vi "Copy To Memory-User.vi"(6 "Select User Trace (1: 1)":u16(ring)=1 items=["1"=1, "2"=2, "3"=3, "4"=4, "5"=5, "6"=6, "7"=7, "8"=8], 7 "Select Current Trace (1: 1)":u16(ring)=1 items=["1"=1, "2"=2, "3"=3, "4"=4, "5"=5, "6"=6, "7"=7, "8"=8], 8 "error in (no error)":errorcluster, 9 "Operation (0: Copy To Memory)":enum16{"Copy To Memory", "Copy To User"}(ring), 10 "Measurement Type (6: Phase Noise)":u16(ring)=6 items=["AM Noise"=1, "Baseband Noise"=2, "Freq/Power"=3, "Spectrum"=4, "Transient"=5, "Phase Noise"=6, "User"=7], 11 "VISA resource name":refnum<visa-resource-name>) -> (0 "error out":errorcluster, 3 "VISA resource name out":refnum<visa-resource-name>)   [LabVIEW 2011, in "Agilent E5052X.lvlib"]
doc: "Copies the selected trace to memory or to the selected user trace."
uses:
  Agilent E5052X.lvlib
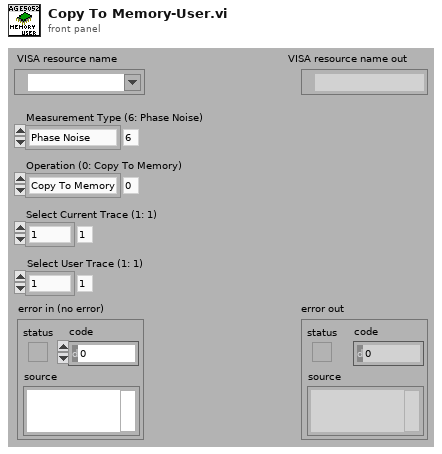
[diagram p1: front panel]
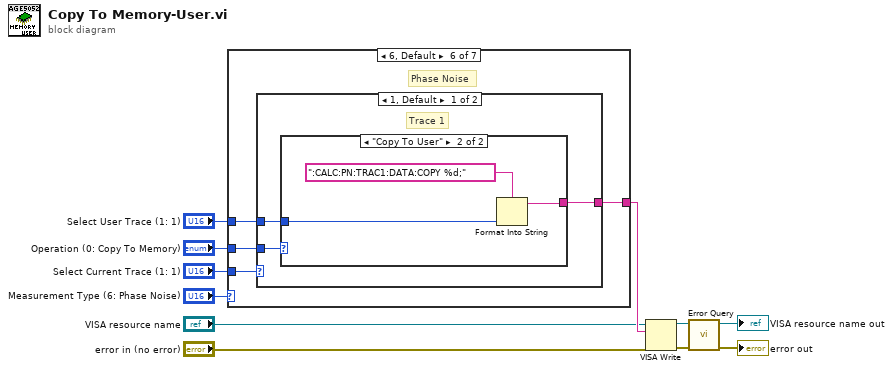
[diagram p0: block diagram]
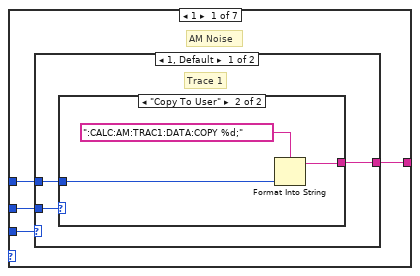
[diagram p2: hidden frame]
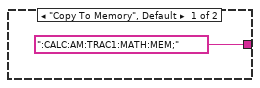
[diagram p3: hidden frame]
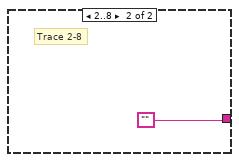
[diagram p4: hidden frame]
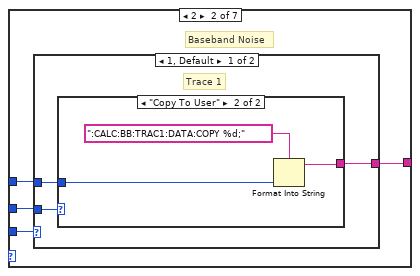
[diagram p5: hidden frame]
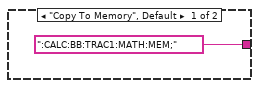
[diagram p6: hidden frame]
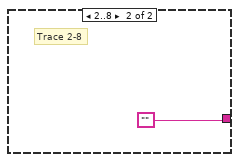
[diagram p7: hidden frame]
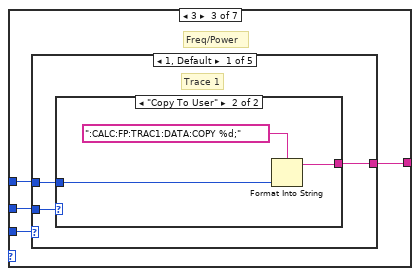
[diagram p8: hidden frame]
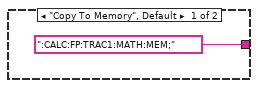
[diagram p9: hidden frame]
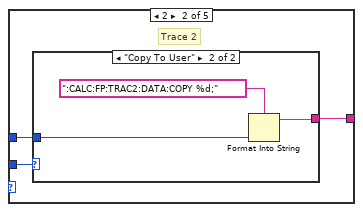
[diagram p10: hidden frame]
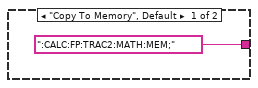
[diagram p11: hidden frame]
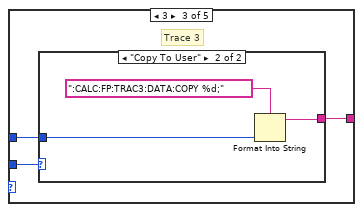
[diagram p12: hidden frame]
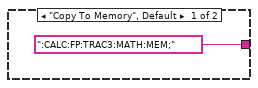
[diagram p13: hidden frame]
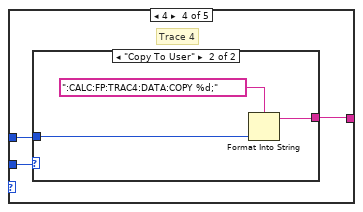
[diagram p14: hidden frame]
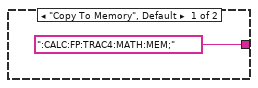
[diagram p15: hidden frame]
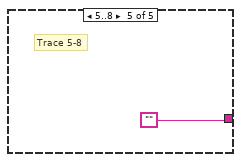
[diagram p16: hidden frame]
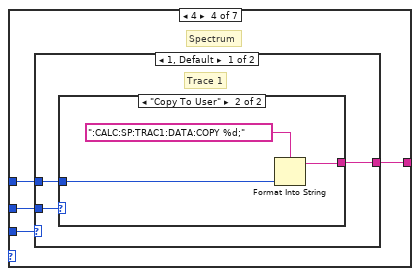
[diagram p17: hidden frame]
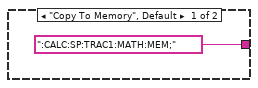
[diagram p18: hidden frame]
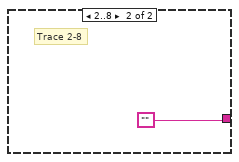
[diagram p19: hidden frame]
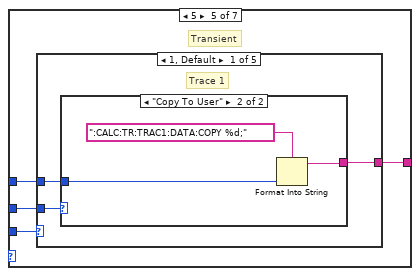
[diagram p20: hidden frame]
diagram:
  n1 = case shown="6, Default" "Measurement Type (6: Phase Noise)" {
    tunnel: "Select Current Trace (1: 1)" -> [w15 w25 w37 w70 w82 w115 w127]
    tunnel: "Operation (0: Copy To Memory)" -> [w14 w26 w38 w71 w83 w116 w128]
    tunnel: "Select User Trace (1: 1)" -> [w13 w27 w39 w72 w84 w117 w129]
    tunnel: [w12 w24 w36 w69 w81 w114 w126] -> w8
    frame 1 {
      # "AM Noise"
      n2 = case shown="1, Default" w15 {
        tunnel: w14 -> [w18 _]
        tunnel: w13 -> [w17 _]
        tunnel: [w16 ""] -> w12
        frame 1, Default {
          # "Trace 1"
          n3 = case shown="\"Copy To User\"" w18 {
            tunnel: [":CALC:AM:TRAC1:MATH:MEM;" w20] -> w16
            tunnel: w17 -> [_ w22]
            frame "Copy To Memory", Default {
            }
            frame "Copy To User" {
              n4 = Format Into String(format string=":CALC:AM:TRAC1:DATA:COPY %d;", w22) -> (resulting string=w20:string)  [unwired: 2 in, 1 out]
            }
          }
        }
        frame 2..8 {
          # "Trace 2-8"
        }
      }
    }
    frame 2 {
      # "Baseband Noise"
      n5 = case shown="1, Default" w25 {
        tunnel: w26 -> [w30 _]
        tunnel: w27 -> [w29 _]
        tunnel: [w28 ""] -> w24
        frame 1, Default {
          # "Trace 1"
          n6 = case shown="\"Copy To User\"" w30 {
            tunnel: [":CALC:BB:TRAC1:MATH:MEM;" w32] -> w28
            tunnel: w29 -> [_ w34]
            frame "Copy To Memory", Default {
            }
            frame "Copy To User" {
              n7 = Format Into String(format string=":CALC:BB:TRAC1:DATA:COPY %d;", w34) -> (resulting string=w32:string)  [unwired: 2 in, 1 out]
            }
          }
        }
        frame 2..8 {
          # "Trace 2-8"
        }
      }
    }
    frame 3 {
      # "Freq/Power"
      n8 = case shown="1, Default" w37 {
        tunnel: w38 -> [w42 w48 w55 w62 _]
        tunnel: w39 -> [w41 w49 w56 w63 _]
        tunnel: [w40 w47 w54 w61 ""] -> w36
        frame 1, Default {
          # "Trace 1"
          n9 = case shown="\"Copy To User\"" w42 {
            tunnel: [":CALC:FP:TRAC1:MATH:MEM;" w44] -> w40
            tunnel: w41 -> [_ w46]
            frame "Copy To Memory", Default {
            }
            frame "Copy To User" {
              n10 = Format Into String(format string=":CALC:FP:TRAC1:DATA:COPY %d;", w46) -> (resulting string=w44:string)  [unwired: 2 in, 1 out]
            }
          }
        }
        frame 2 {
          # "Trace 2"
          n11 = case shown="\"Copy To User\"" w48 {
            tunnel: [":CALC:FP:TRAC2:MATH:MEM;" w51] -> w47
            tunnel: w49 -> [_ w53]
            frame "Copy To Memory", Default {
            }
            frame "Copy To User" {
              n12 = Format Into String(format string=":CALC:FP:TRAC2:DATA:COPY %d;", w53) -> (resulting string=w51:string)  [unwired: 2 in, 1 out]
            }
          }
        }
        frame 3 {
          # "Trace 3"
          n13 = case shown="\"Copy To User\"" w55 {
            tunnel: [":CALC:FP:TRAC3:MATH:MEM;" w58] -> w54
            tunnel: w56 -> [_ w60]
            frame "Copy To Memory", Default {
            }
            frame "Copy To User" {
              n14 = Format Into String(format string=":CALC:FP:TRAC3:DATA:COPY %d;", w60) -> (resulting string=w58:string)  [unwired: 2 in, 1 out]
            }
          }
        }
        frame 4 {
          # "Trace 4"
          n15 = case shown="\"Copy To User\"" w62 {
            tunnel: [":CALC:FP:TRAC4:MATH:MEM;" w65] -> w61
            tunnel: w63 -> [_ w67]
            frame "Copy To Memory", Default {
            }
            frame "Copy To User" {
              n16 = Format Into String(format string=":CALC:FP:TRAC4:DATA:COPY %d;", w67) -> (resulting string=w65:string)  [unwired: 2 in, 1 out]
            }
          }
        }
        frame 5..8 {
          # "Trace 5-8"
        }
      }
    }
    frame 4 {
      # "Spectrum"
      n17 = case shown="1, Default" w70 {
        tunnel: w71 -> [w75 _]
        tunnel: w72 -> [w74 _]
        tunnel: [w73 ""] -> w69
        frame 1, Default {
          # "Trace 1"
          n18 = case shown="\"Copy To User\"" w75 {
            tunnel: [":CALC:SP:TRAC1:MATH:MEM;" w77] -> w73
            tunnel: w74 -> [_ w79]
            frame "Copy To Memory", Default {
            }
            frame "Copy To User" {
              n19 = Format Into String(format string=":CALC:SP:TRAC1:DATA:COPY %d;", w79) -> (resulting string=w77:string)  [unwired: 2 in, 1 out]
            }
          }
        }
        frame 2..8 {
          # "Trace 2-8"
        }
      }
    }
    frame 5 {
      # "Transient"
      n20 = case shown="1, Default" w82 {
        tunnel: w83 -> [w87 w93 w100 w107 _]
        tunnel: w84 -> [w86 w94 w101 w108 _]
        tunnel: [w85 w92 w99 w106 ""] -> w81
        frame 1, Default {
          # "Trace 1"
          n21 = case shown="\"Copy To User\"" w87 {
            tunnel: [":CALC:TR:TRAC1:MATH:MEM;" w89] -> w85
            tunnel: w86 -> [_ w91]
            frame "Copy To Memory", Default {
            }
            frame "Copy To User" {
              n22 = Format Into String(format string=":CALC:TR:TRAC1:DATA:COPY %d;", w91) -> (resulting string=w89:string)  [unwired: 2 in, 1 out]
            }
          }
        }
        frame 2 {
          # "Trace 2"
          n23 = case shown="\"Copy To User\"" w93 {
            tunnel: [":CALC:TR:TRAC2:MATH:MEM;" w96] -> w92
            tunnel: w94 -> [_ w98]
            frame "Copy To Memory", Default {
            }
            frame "Copy To User" {
              n24 = Format Into String(format string=":CALC:TR:TRAC2:DATA:COPY %d;", w98) -> (resulting string=w96:string)  [unwired: 2 in, 1 out]
            }
          }
        }
        frame 3 {
          # "Trace 3"
          n25 = case shown="\"Copy To User\"" w100 {
            tunnel: [":CALC:TR:TRAC3:MATH:MEM;" w103] -> w99
            tunnel: w101 -> [_ w105]
            frame "Copy To Memory", Default {
            }
            frame "Copy To User" {
              n26 = Format Into String(format string=":CALC:TR:TRAC3:DATA:COPY %d;", w105) -> (resulting string=w103:string)  [unwired: 2 in, 1 out]
            }
          }
        }
        frame 4 {
          # "Trace 4"
          n27 = case shown="\"Copy To User\"" w107 {
            tunnel: [":CALC:TR:TRAC4:MATH:MEM;" w110] -> w106
            tunnel: w108 -> [_ w112]
            frame "Copy To Memory", Default {
            }
            frame "Copy To User" {
              n28 = Format Into String(format string=":CALC:TR:TRAC4:DATA:COPY %d;", w112) -> (resulting string=w110:string)  [unwired: 2 in, 1 out]
            }
          }
        }
        frame 5..8 {
          # "Trace 5-8"
        }
      }
    }
    frame 6, Default {
      # "Phase Noise"
      n29 = case shown="1, Default" w115 {
        tunnel: w116 -> [w120 _]
        tunnel: w117 -> [w119 _]
        tunnel: [w118 ""] -> w114
        frame 1, Default {
          # "Trace 1"
          n30 = case shown="\"Copy To User\"" w120 {
            tunnel: [":CALC:PN:TRAC1:MATH:MEM;" w122] -> w118
            tunnel: w119 -> [_ w124]
            frame "Copy To Memory", Default {
            }
            frame "Copy To User" {
              n31 = Format Into String(format string=":CALC:PN:TRAC1:DATA:COPY %d;", w124) -> (resulting string=w122:string)  [unwired: 2 in, 1 out]
            }
          }
        }
        frame 2..8 {
          # "Trace 2-8"
        }
      }
    }
    frame 7 {
      # "User"
      n32 = case shown="1, Default" w127 {
        tunnel: w128 -> [w132 w138 w145 w152 w159 w166 w173 w180]
        tunnel: w129 -> [w131 w139 w146 w153 w160 w167 w174 w181]
        tunnel: [w130 w137 w144 w151 w158 w165 w172 w179] -> w126
        frame 1, Default {
          # "Trace 1"
          n33 = case shown="\"Copy To User\"" w132 {
            tunnel: [":CALC:USER:TRAC1:MATH:MEM;" w134] -> w130
            tunnel: w131 -> [_ w136]
            frame "Copy To Memory", Default {
            }
            frame "Copy To User" {
              n34 = Format Into String(format string=":CALC:USER:TRAC1:DATA:COPY %d;", w136) -> (resulting string=w134:string)  [unwired: 2 in, 1 out]
            }
          }
        }
        frame 2 {
          # "Trace 2"
          n35 = case shown="\"Copy To User\"" w138 {
            tunnel: [":CALC:USER:TRAC2:MATH:MEM;" w141] -> w137
            tunnel: w139 -> [_ w143]
            frame "Copy To Memory", Default {
            }
            frame "Copy To User" {
              n36 = Format Into String(format string=":CALC:USER:TRAC2:DATA:COPY %d;", w143) -> (resulting string=w141:string)  [unwired: 2 in, 1 out]
            }
          }
        }
        frame 3 {
          # "Trace 3"
          n37 = case shown="\"Copy To User\"" w145 {
            tunnel: [":CALC:USER:TRAC3:MATH:MEM;" w148] -> w144
            tunnel: w146 -> [_ w150]
            frame "Copy To Memory", Default {
            }
            frame "Copy To User" {
              n38 = Format Into String(format string=":CALC:USER:TRAC3:DATA:COPY %d;", w150) -> (resulting string=w148:string)  [unwired: 2 in, 1 out]
            }
          }
        }
        frame 4 {
          # "Trace 4"
          n39 = case shown="\"Copy To User\"" w152 {
            tunnel: [":CALC:USER:TRAC4:MATH:MEM;" w155] -> w151
            tunnel: w153 -> [_ w157]
            frame "Copy To Memory", Default {
            }
            frame "Copy To User" {
              n40 = Format Into String(format string=":CALC:USER:TRAC4:DATA:COPY %d;", w157) -> (resulting string=w155:string)  [unwired: 2 in, 1 out]
            }
          }
        }
        frame 5 {
          # "Trace 5"
          n41 = case shown="\"Copy To User\"" w159 {
            tunnel: [":CALC:USER:TRAC5:MATH:MEM;" w162] -> w158
            tunnel: w160 -> [_ w164]
            frame "Copy To Memory", Default {
            }
            frame "Copy To User" {
              n42 = Format Into String(format string=":CALC:USER:TRAC5:DATA:COPY %d;", w164) -> (resulting string=w162:string)  [unwired: 2 in, 1 out]
            }
          }
        }
        frame 6 {
          # "Trace 6"
          n43 = case shown="\"Copy To User\"" w166 {
            tunnel: [":CALC:USER:TRAC6:MATH:MEM;" w169] -> w165
            tunnel: w167 -> [_ w171]
            frame "Copy To Memory", Default {
            }
            frame "Copy To User" {
              n44 = Format Into String(format string=":CALC:USER:TRAC6:DATA:COPY %d;", w171) -> (resulting string=w169:string)  [unwired: 2 in, 1 out]
            }
          }
        }
        frame 7 {
          # "Trace 7"
          n45 = case shown="\"Copy To User\"" w173 {
            tunnel: [":CALC:USER:TRAC7:MATH:MEM;" w176] -> w172
            tunnel: w174 -> [_ w178]
            frame "Copy To Memory", Default {
            }
            frame "Copy To User" {
              n46 = Format Into String(format string=":CALC:USER:TRAC7:DATA:COPY %d;", w178) -> (resulting string=w176:string)  [unwired: 2 in, 1 out]
            }
          }
        }
        frame 8 {
          # "Trace 8"
          n47 = case shown="\"Copy To User\"" w180 {
            tunnel: [":CALC:USER:TRAC8:MATH:MEM;" w183] -> w179
            tunnel: w181 -> [_ w185]
            frame "Copy To Memory", Default {
            }
            frame "Copy To User" {
              n48 = Format Into String(format string=":CALC:USER:TRAC8:DATA:COPY %d;", w185) -> (resulting string=w183:string)  [unwired: 2 in, 1 out]
            }
          }
        }
      }
    }
  }
  n49 = VISA Write(VISA resource name="VISA resource name", write buffer=w8, error in (no error)="error in (no error)") -> (VISA resource name out=w7:refnum<visa-resource-name>, error out=w6:errorcluster)  [unwired: 1 out]
  n50 = call "Error Query.vi"("error in (no error)"=w6, "VISA resource name"=w7) -> ("error out"=→"error out":errorcluster, "VISA resource name out"=→"VISA resource name out":refnum<visa-resource-name>)  [unwired: 6 in, 2 out]
